vi "contrast continuous move V1.vi"(8 "error in (no error)":errorcluster, 11 "?":T2[](array[typedef])) -> (0 "error out":errorcluster)   [LabVIEW 2019]
uses:
  ctl/continued move array-V2.ctl
  <vilib>/platform/TimedLoop/XDataNode/XDataNode.xnode
  <vilib>/Platform/TimedLoop/XDataNode/nitl_modes.ctl
  <vilib>/Platform/TimedLoop/XDataNode/XDNodeRunTimeDep.lvlib
  <vilib>/Platform/TimedLoop/XDataNode/wakeup.ctl
  <vilib>/Platform/TimedLoop/XDataNode/timing_clust.ctl
  gyro/BNO055/class/angle Converter.lvclass
  <vilib>/addons/control/pid/NI_PID_pid.lvlib
  <vilib>/addons/control/pid/pid.llb/PID (DBL).vi
panel:
  out "result":bool
  out "Waveform Chart":T1(graph)
  out "i 2":i32
  out "i":i32
  in  "stop":bool
  out "s? t:f 2":i32
  out "s? t:f":i32
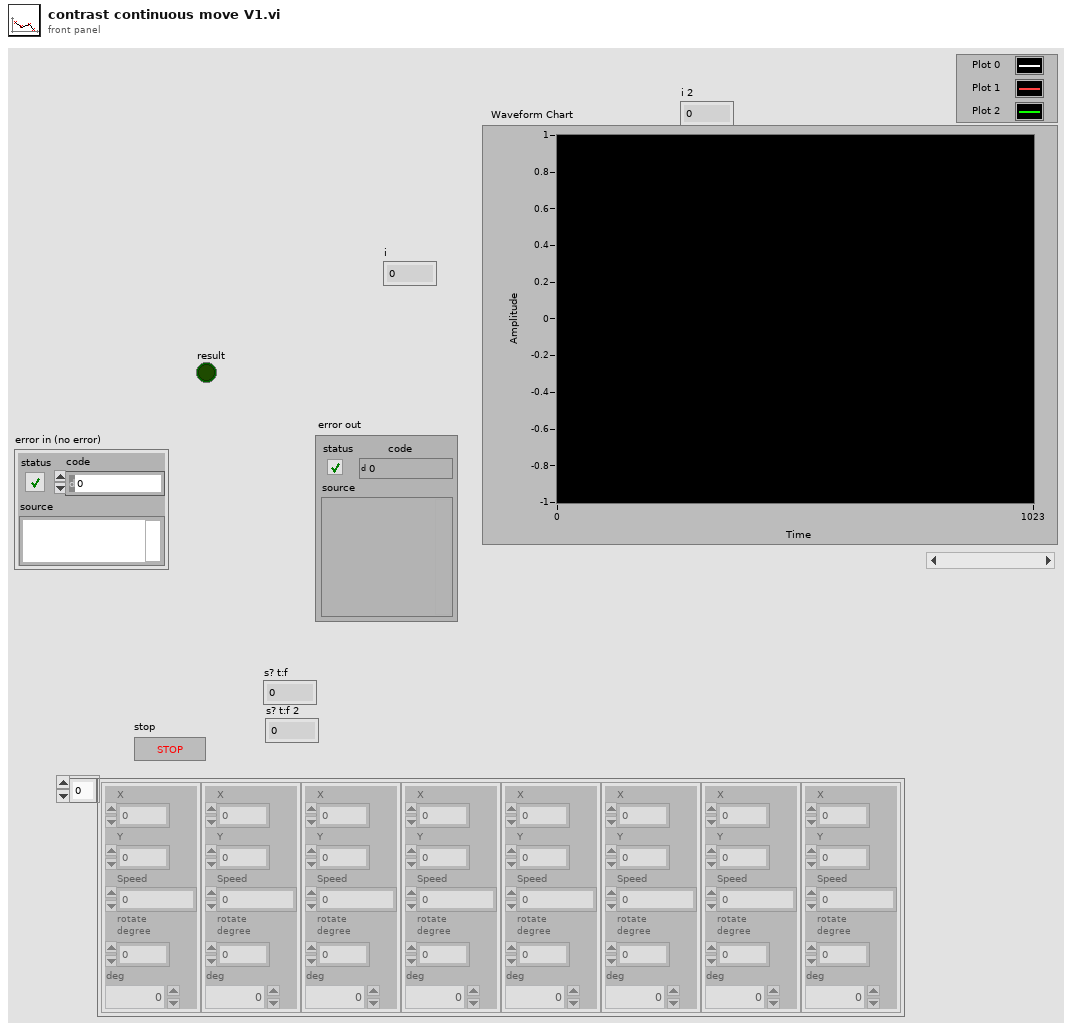
[diagram p1: front panel]
types:
  T1 = cluster{"out":dbl, "angle out":dbl, "upper limit":dbl}
  T2 = typedef "continued move array-V2.ctl" = cluster{"X":dbl, "Y":dbl, "Speed":dbl, "rotate\ndegree":dbl, "deg":dbl}
  T3 = typedef "XDNodeRunTimeDep.lvlib/timing_clust.ctl" = cluster{"Expected End [f-1]":u64, "Actual End [f-1]":u64, "Finished Late? [f-1]":bool, "Expected End [i-1]":u64, "Actual End [i-1]":u64, "Finished Late? [i-1]":bool, "Expected Start [i]":u64, "Actual Start [i]":u64, "Expected Start [f]":u64, "Actual Start [f]":u64, "Source Name":string, "Structure Name":string, "Period":i64, "Deadline":i64, "Offset":i64, "Start":i64, "Priority":i32, "Timeout":i32, "Mode":T4, "Wakeup Reason":T5, "Error":errorcluster, "Source Type":string, "Secondary Source Type":string, "Global End Time":u64, "Global Start Time":u64, "Frame Duration":u64, "Iteration Duration":u64, "Assigned CPU":i32, "I/O Scan Engine Mode":u32}
  T4 = typedef "XDNodeRunTimeDep.lvlib/nitl_modes.ctl" = enum32{"No Change", "Process missed periods, maintain original phase", "Discard missed periods, maintain original phase", "Process missed periods, ignore original phase", "Discard missed periods, ignore original phase"}
  T5 = typedef "XDNodeRunTimeDep.lvlib/wakeup.ctl" = enum32{"Normal", "Aborted", "Asynchronous wakeup", "Timing source error", "Timed loop error", "Timeout"}
  T6 = cluster{"output":dbl, "angle out":dbl, "upper limit":dbl}
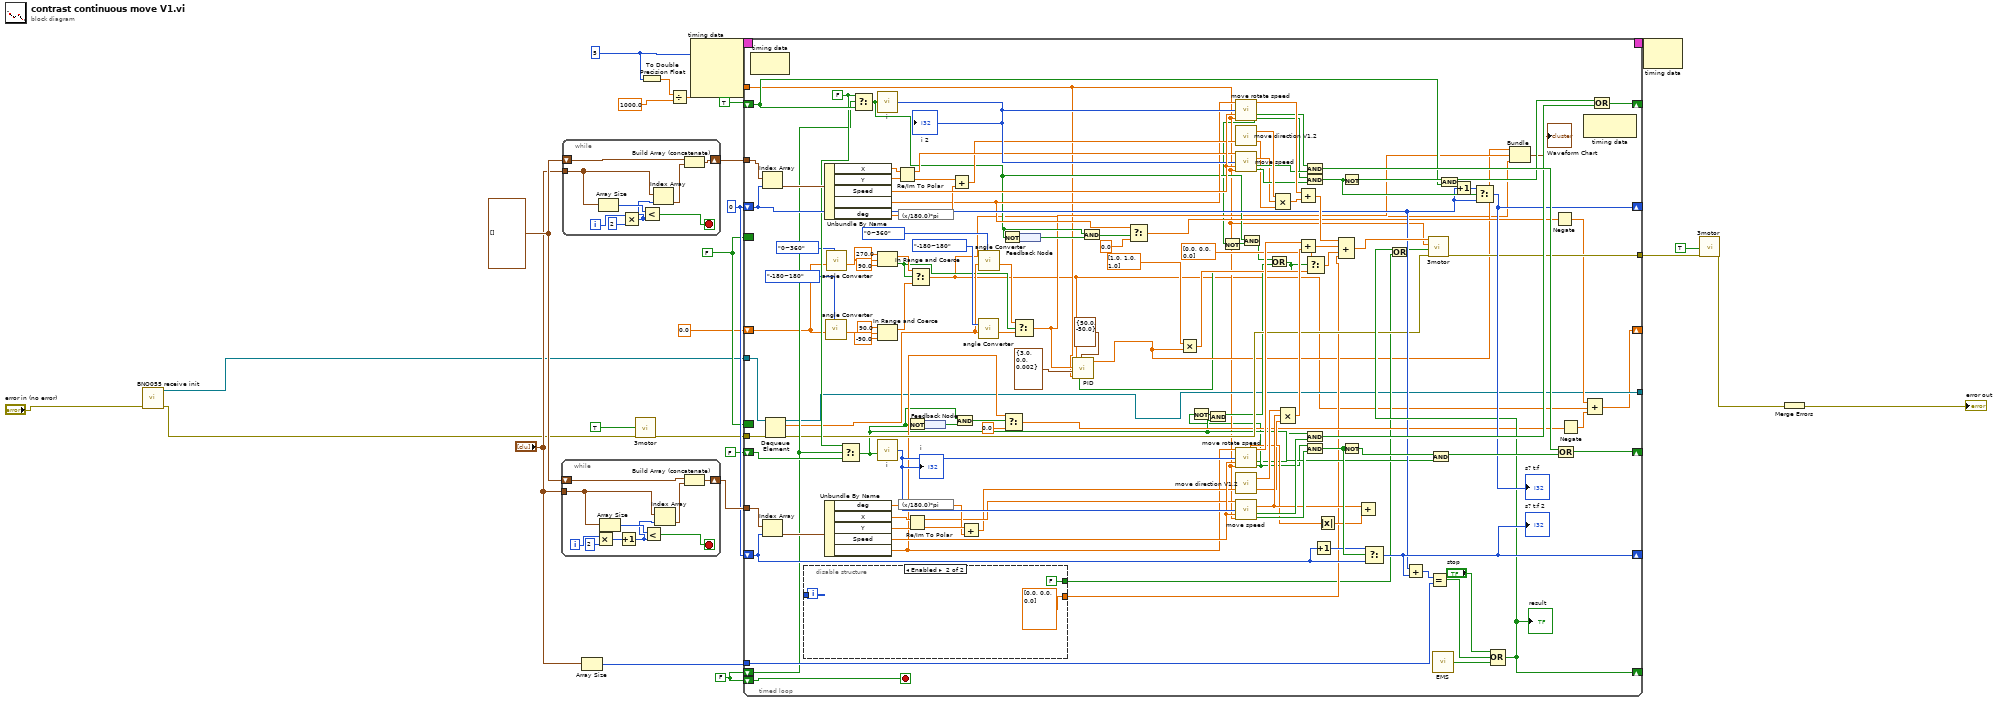
[diagram p0: block diagram]
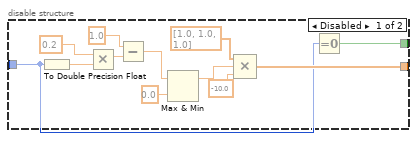
[diagram p2: hidden frame]
diagram:
  w7 = FALSE
  w9 = FALSE
  w20 = i64 5 ("Period")
  w15 = 0
  w26 = T2[] []
  n1 = call "BNO055 receive init.vi"("error in (no error)"="error in (no error)") -> ("error out"=w3:errorcluster, "rt fifo out"=w4:refnum<k33>)  [unwired: 8 in, 1 out]
  n2 = while {
    tunnel: "?" -> [w31]
    shift-right: [w30] -> w16
    shift-left: w26 -> [w29]
    i -> [w36]
    stop <- w33 stop-if-true
    n3 = Multiply(x=w36, y=2) -> (x*y=w32:i32)
    n4 = Array Size(array=w31) -> (size(s)=w34:i32)
    n5 = Increment(x=w32) -> (x+1=w27:i32)
    n6 = Less?(x=w34, y=w27) -> (x < y?=w33:bool)
    n7 = Index Array(array=w31, index=w27) -> (element=w28:T2)
    n8 = Build Array (concatenate)(w29, w28) -> (w30:T2[])
  }
  n9 = while {
    tunnel: "?" -> [w40]
    shift-right: [w39] -> w22
    shift-left: w26 -> [w38]
    i -> [w45]
    stop <- w42 stop-if-true
    n10 = Array Size(array=w40) -> (size(s)=w43:i32)
    n11 = Multiply(x=w45, y=2) -> (x*y=w41:i32)
    n12 = Less?(x=w43, y=w41) -> (x < y?=w42:bool)
    n13 = Index Array(array=w40, index=w41) -> (element=w37:T2)
    n14 = Build Array (concatenate)(w38, w37) -> (w39:T2[])
  }
  n15 = Array Size(array="?") -> (size(s)=w23:i32)
  n16 = call "3motor.vi"("error in (no error)"=w3, "Reset"=TRUE) -> ("error out"=w6:errorcluster)  [unwired: 8 in, 1 out]
  n17 = To Double Precision Float(number=w20) -> (double precision float=w19:dbl)
  n18 = Divide(x=w19, y=1000.0) -> (x/y=w17:dbl)
  n19 = node-c288(w20) -> (w25:T3)  [unwired: 3 in]
  n20 = timed-loop {
    timing: w25 -> [_]
    timing-out: [_] -> w24
    tunnel: w23 -> [w143]
    shift-right: [w165] -> _
    shift-left: TRUE -> [w130]
    shift-right: [w146] -> _
    shift-left: w15 -> [w128]
    tunnel: w17 -> [w51]
    shift-right: [w162] -> _
    shift-left: FALSE -> [w127]
    shift-right: [w145] -> _
    shift-left: w15 -> [w147]
    tunnel: w16 -> [w170]
    tunnel: w22 -> [w129]
    tunnel: w6 -> [w94]
    tunnel: [w137] -> w12
    shift-right: [w131] -> _
    shift-left: w9 -> [w125]
    shift-left: w9 -> [w124]
    border: w7 -> [_]
    border: w7 -> [_]
    tunnel: w4 -> [w60]
    tunnel: [w59] -> _
    shift-right: [w58] -> _
    shift-left: 0.0 -> [w57]
    i -> [w62]
    stop <- w124 stop-if-true
    w126 = FALSE
    n21 = node-c288() -> ()  [unwired: 1 in, 1 out]
    n22 = Index Array(array=w129, index=w128) -> (element=w176:T2)
    n23 = Index Array(array=w170, index=w147) -> (element=w171:T2)
    n24 = Dequeue Element(queue=w60, error in (no error)=w94) -> (queue out=w59:refnum<queue>, element=w92:dbl, error out=w93:errorcluster)  [unwired: 1 in, 1 out]
    n25 = disable-structure shown="Enabled" {
      disable-tunnel: [w180 dbl[] [0.0, 0.0, 0.0]] -> w64
      disable-tunnel: w62 -> [w178 _]
      disable-tunnel: [w177 FALSE] -> w61
      frame Disabled {
        n26 = To Double Precision Float(number=w178) -> (double precision float=w188:dbl)
        n27 = Multiply(x=0.2, y=w188) -> (x*y=w187:dbl)
        n28 = Subtract(x=1.0, y=w187) -> (x-y=w184:dbl)
        n29 = Max & Min(x=w184, y=0.0) -> (max(x,y)=w181:dbl)  [unwired: 1 out]
        n30 = Compound Arithmetic op=MULTIPLY(dbl[] [1.0, 1.0, 1.0], w181, -10.0) -> (w180:dbl[])
        n31 = Equal To 0?(x=w178) -> (x = 0?=w177:bool)
      }
      frame Enabled {
      }
    }
    n32 = Unbundle By Name(w176) -> ("X"=w116:dbl, "Y"=w115:dbl, "Speed"=w175:dbl, "rotate\ndegree"=w76:dbl, "deg"=w121:dbl)
    n33 = Unbundle By Name(w171) -> ("deg"=w118:dbl, "X"=w114:dbl, "Y"=w113:dbl, "Speed"=w172:dbl, "rotate\ndegree"=w74:dbl)
    n34 = call "angle Converter.vi"("select"=enum16{"-180~180", "0~360"}."-180~180", "input angle"=w57) -> ("angle out"=w99:dbl)  [unwired: 9 in]
    n35 = call "angle Converter.vi"("select"=enum16{"-180~180", "0~360"}."0~360", "input angle"=w57) -> ("angle out"=w102:dbl)  [unwired: 9 in]
    n36 = Select(t=w126, s=w125, f=w127) -> (s? t:f=w69:bool)
    n37 = Select(t=w126, s=w125, f=w130) -> (s? t:f=w70:bool)
    n38 = call "i.vi"("start"=w70) -> ("i"=w174:i32)
    "i 2" <- w174
    n39 = In Range and Coerce(upper limit=270.0, x=w102, lower limit=90.0) -> (coerced(x)=w98:dbl, In Range?=w89:bool)
    n40 = In Range and Coerce(upper limit=90.0, x=w99, lower limit=-90.0) -> (coerced(x)=w97:dbl)  [unwired: 1 out]
    n41 = call "i.vi"("start"=w69) -> ("i"=w173:i32)
    "i" <- w173
    n42 = Re/Im To Polar(2:w115, 3:w116) -> (0:w122:dbl, 1:w109:dbl)
    n43 = expression code="(x/180.0)*pi" ("degrees to radians")(w121) -> (w120:dbl)
    n44 = expression code="(x/180.0)*pi" ("degrees to radians")(w118) -> (w117:dbl)
    n45 = Not(x=w69) -> (.not. x?=w68:bool)
    n46 = Re/Im To Polar(2:w113, 3:w114) -> (0:w119:dbl, 1:w110:dbl)
    n47 = Select(t=w98, s=w89, f=w97) -> (s? t:f=w50:dbl)
    n48 = feedback #1() -> (w73:bool)
    n49 = feedback-in #1(w68) -> ()
    n50 = Add(x=w122, y=w120) -> (x+y=w108:dbl)
    n51 = And(x=w69, y=w73) -> (x .and. y?=w72:bool)
    n52 = Add(x=w119, y=w117) -> (x+y=w107:dbl)
    n53 = call "angle Converter.vi"("select"=enum16{"-180~180", "0~360"}."-180~180", "input angle"=w92) -> ("angle out"=w90:dbl)  [unwired: 9 in]
    n54 = call "angle Converter.vi"("select"=enum16{"-180~180", "0~360"}."0~360", "input angle"=w92) -> ("angle out"=w91:dbl)  [unwired: 9 in]
    n55 = Not(x=w70) -> (.not. x?=w67:bool)
    n56 = Select(t=w74, s=w72, f=0.0) -> (s? t:f=w80:dbl)
    n57 = Select(t=w91, s=w89, f=w90) -> (s? t:f=w56:dbl)
    n58 = feedback #2() -> (w79:bool)
    n59 = feedback-in #2(w67) -> ()
    n60 = And(x=w70, y=w79) -> (x .and. y?=w78:bool)
    n61 = Select(t=w76, s=w78, f=0.0) -> (s? t:f=w75:dbl)
    n62 = call "move rotate speed.vi"("rotate degree"=w76, "i"=w174, "speed"=w175, "dt(s)"=w51) -> ("speed out"=w167:dbl[], "t2?"=w46:bool, "complet?"=w48:bool)  [unwired: 5 in, 4 out]
    n63 = Not(x=w48) -> (.not. x?=w85:bool)
    n64 = call "move direction V1.2.vi"("theta"=w108) -> ("max value"=w111:dbl, "out array"=w169:dbl[])  [unwired: 1 in]
    n65 = call "move speed.vi"("X"=w109, "i"=w174, "speed"=w175, "dt(s)"=w51) -> ("speed out"=w132:dbl, "t2?"=w160:bool, "complet?"=w166:bool)  [unwired: 7 in, 2 out]
    n66 = call "move rotate speed.vi"("rotate degree"=w74, "i"=w173, "speed"=w172, "dt(s)"=w51) -> ("speed"=w134:dbl, "speed out"=w154:dbl[], "t2?"=w47:bool, "complet?"=w49:bool)  [unwired: 5 in, 3 out]
    n67 = Not(x=w49) -> (.not. x?=w84:bool)
    n68 = And(x=w84, y=w69) -> (x .and. y?=w82:bool)
    n69 = call "move direction V1.2.vi"("theta"=w107) -> ("max value"=w112:dbl, "out array"=w156:dbl[])  [unwired: 1 in]
    n70 = call "move speed.vi"("X"=w110, "i"=w173, "speed"=w172, "dt(s)"=w51) -> ("speed out"=w136:dbl, "t2?"=w158:bool, "complet?"=w163:bool)  [unwired: 7 in, 2 out]
    n71 = And(x=w70, y=w85) -> (x .and. y?=w81:bool)
    n72 = Or(x=w81, y=w82) -> (x .or. y?=w52:bool)
    n73 = call-poly <vilib>:"PID.vi"("reinitialize? (F)"=w52, "output range"=cluster{"output high":dbl, "output low":dbl} {"output high"=50.0, "output low"=-50.0}, "dt (s)"=w51, "PID gains"=cluster{"Kp":dbl, "Ki":dbl, "Kd":dbl} {"Kp"=3.0, "Ki"=0.0, "Kd"=0.002} ("PID"), "process variable"=w56, "setpoint"=w50) -> ("output"=w53:dbl)  [unwired: 4 in, 1 out]
    n74 = Multiply(x=dbl[] [1.0, 1.0, 1.0], y=w53) -> (x*y=w87:dbl[])
    n75 = Compound Arithmetic op=MULTIPLY(w169, w132, w111) -> (w168:dbl[])
    n76 = Compound Arithmetic op=MULTIPLY(w156, w136, w112) -> (w155:dbl[])
    n77 = Add(x=w167, y=w168) -> (x+y=w139:dbl[])
    n78 = Add(x=w154, y=w155) -> (x+y=w140:dbl[])
    n79 = And(x=w46, y=w160) -> (x .and. y?=w159:bool)
    n80 = And(x=w48, y=w166) -> (x .and. y?=w151:bool)
    n81 = Select(t=dbl[] [0.0, 0.0, 0.0], s=w52, f=w87) -> (s? t:f=w86:dbl[])
    n82 = And(x=w47, y=w158) -> (x .and. y?=w157:bool)
    n83 = And(x=w49, y=w163) -> (x .and. y?=w149:bool)
    n84 = Increment(x=w147) -> (x+1=w148:i32)
    n85 = Absolute Value(x=w134) -> (abs(x)=w133:dbl)
    n86 = Compound Arithmetic op=ADD(w139, w140, w86, w64) -> (w138:dbl[])
    n87 = Not(x=w151) -> (.not. x?=w164:bool)
    n88 = Not(x=w149) -> (.not. x?=w161:bool)
    n89 = Add(x=w136, y=w133) -> ()  [unwired: 1 out]
    n90 = Select(t=w148, s=w149, f=w147) -> (s? t:f=w145:i32)
    "s? t:f 2" <- w145
    n91 = Add(x=w128, y=w145) -> (x+y=w144:i32)
    n92 = Equal?(x=w144, y=w143) -> (x = y?=w142:bool)
    n93 = And(x=w161, y=w69) -> (x .and. y?=w152:bool)
    n94 = call "EMS.vi"() -> ("A/DIO4 (Pin 19)"=w123:bool)
    n95 = And(x=w164, y=w130) -> (x .and. y?=w153:bool)
    n96 = Increment(x=w128) -> (x+1=w150:i32)
    n97 = Select(t=w150, s=w151, f=w128) -> (s? t:f=w146:i32)
    "s? t:f" <- w146
    n98 = Compound Arithmetic op=OR("stop", w142, w123) -> (w131:bool)
    "result" <- w131
    n99 = Or(x=w131, y=w61) -> (x .or. y?=w63:bool)
    n100 = call "3motor.vi"("error in (no error)"=w93, "Reset"=w63, "dt(s)"=w51, "Motor speed"=w138) -> ("error out"=w137:errorcluster)  [unwired: 6 in, 1 out]
    n101 = Bundle("output"=w53, "angle out"=w56, "upper limit"=w50) -> (→"Waveform Chart":T6)  [unwired: 1 in]
    n102 = Negate(x=w75) -> (-x=w65:dbl)
    n103 = Compound Arithmetic op=OR(w159, w152) -> (w162:bool)
    n104 = Negate(x=w80) -> (-x=w66:dbl)
    n105 = node-c288() -> ()  [unwired: 1 in, 1 out]
    n106 = Compound Arithmetic op=ADD(w65, w50, w66) -> (w58:dbl)
    n107 = Compound Arithmetic op=OR(w153, w157) -> (w165:bool)
  }
  n108 = node-c288(w24) -> ()  [unwired: 1 out]
  n109 = call "3motor.vi"("error in (no error)"=w12, "Reset"=TRUE) -> ("error out"=w8:errorcluster)  [unwired: 8 in, 1 out]
  n110 = Merge Errors(w8) -> (→"error out":errorcluster)
